vi "Relink Test Executive.vi"(6 "File":path, 7 "Persistence in":refnum<class "IPersist.lvclass">, 8 "error in (no error)":errorcluster, 9 "Compatibility Helper":refnum<class "ICompatibility Helper.lvclass">, 10 "Path Builder":refnum<class "IPath Builder.lvclass">, 11 "Test Executive":refnum<class "ITest Executive.lvclass">) -> (0 "error out":errorcluster, 1 "Return":string, 3 "Test Executive Ref out":refnum<data-value>, 5 "Root ID":string)   [LabVIEW 2020, in "Test Executive.lvlib" / "TestExecutive Ref.lvclass"]
uses:
  <vilib>/gpm_packages/@cs/test-executive/Source/Test Executive/TestExecutive Ref/TestExecutive Ref.lvclass
  <vilib>/gpm_packages/@cs/test-executive/Source/Test Executive/ITestExecutive/ITest Executive.lvclass
  <vilib>/gpm_packages/@cs/persistence/source/IPersist/IPersist.lvclass
  <vilib>/gpm_packages/@cs/test-executive/Source/Path Builder/IPath Builder/IPath Builder.lvclass
  <vilib>/gpm_packages/@cs/test-executive/Source/Compatibility Helper/ICompatibility Helper.lvclass
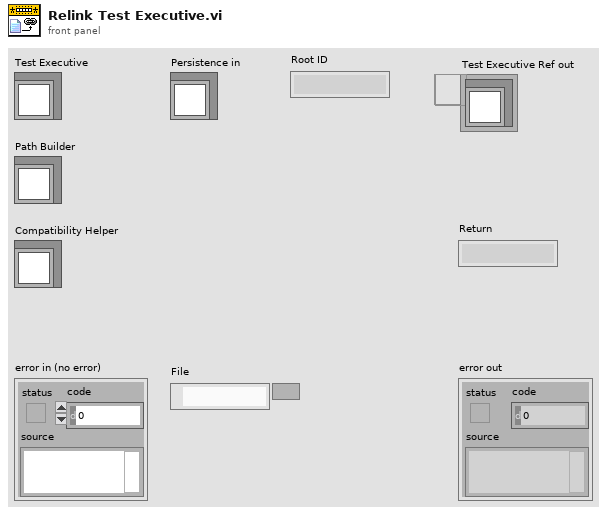
[diagram p1: front panel]
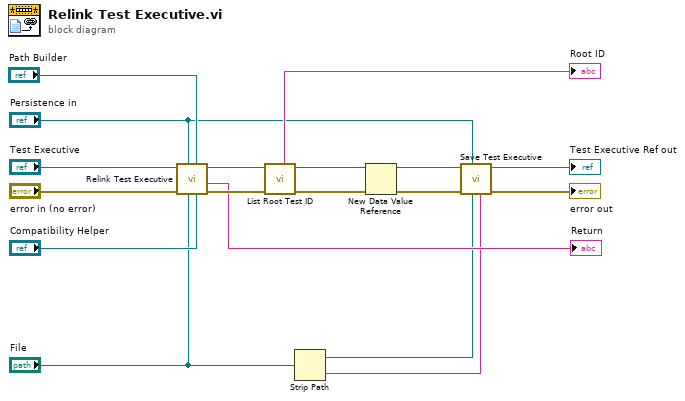
[diagram p0: block diagram]
diagram:
  n1 = call-dynamic "Relink Test Executive.vi"("Compatibility Helper"="Compatibility Helper", "Path Builder"="Path Builder", "File Path"="File", "Persistence in"="Persistence in", "error in (no error)"="error in (no error)", "ITest Executive in"="Test Executive") -> ("error out"=w14:errorcluster, "Return"=→"Return":string, "ITest Executive out"=w16:refnum<class "ITest Executive.lvclass">)  [unwired: 3 in]
  n2 = call-dynamic "List Root Test ID.vi"("error in (no error)"=w14, "ITest Executive in"=w16) -> ("error out"=w13:errorcluster, "ITest Executive out"=w15:refnum<class "ITest Executive.lvclass">, "Root ID"=→"Root ID":string)  [unwired: 5 in, 2 out]
  n3 = Strip Path(path="File") -> (stripped path=w2:path, name=w1:string)
  n4 = New Data Value Reference(data value=w15, error in=w13) -> (data value reference=w8:refnum<data-value>, error out=w6:errorcluster)
  n5 = call <vilib>:"Save Test Executive.vi"("File Name"=w1, "Folder"=w2, "Persistence in"="Persistence in", "error in (no error)"=w6, "Test Executive Ref"=w8) -> ("error out"=→"error out":errorcluster, "Test Executive Ref out"=→"Test Executive Ref out":refnum<data-value>)  [unwired: 5 in]
